vi "Select Item Value.vi"(7 "Section Name":string, 8 "error in (no error)":errorcluster, 10 "Key Name":string, 11 "ODBC-Interface in":refnum<class "ODBC-Interface.lvclass">) -> (0 "error out":errorcluster, 1 "Value":variant, 2 "found":bool, 3 "ODBC-Interface out":refnum<class "ODBC-Interface.lvclass">)   [LabVIEW 2012, in "DB-Configuration.lvlib" / "ODBC-Interface.lvclass"]
doc: "Read item value from database."
uses:
  ODBC-Interface.lvclass
  ODBC-Interface.lvclass/ODBC-Interface.ctl
  <vilib>/addons/database/Connection.llb/Conn Execute.vi
  <vilib>/addons/database/Recordset.llb/Rec Fetch Recordset Data (R).vi
  <vilib>/addons/database/Recordset.llb/Rec Destroy - Connection.vi
  DB-Configuration.lvlib
  <vilib>/addons/database/NI_Database_API.lvlib
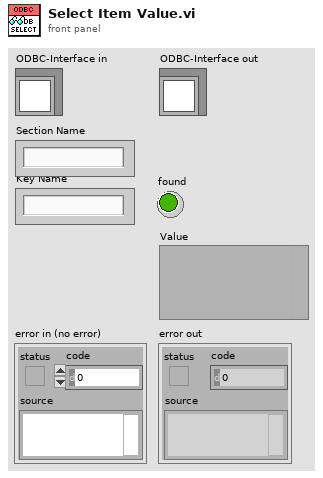
[diagram p1: front panel]
types:
  T1 = typedef "NI_Database_API.lvlib/Conn ObjectReference.ctl" = refnum<k1>
  T2 = typedef "NI_Database_API.lvlib/Rec ObjectReference.ctl" = refnum<k1>
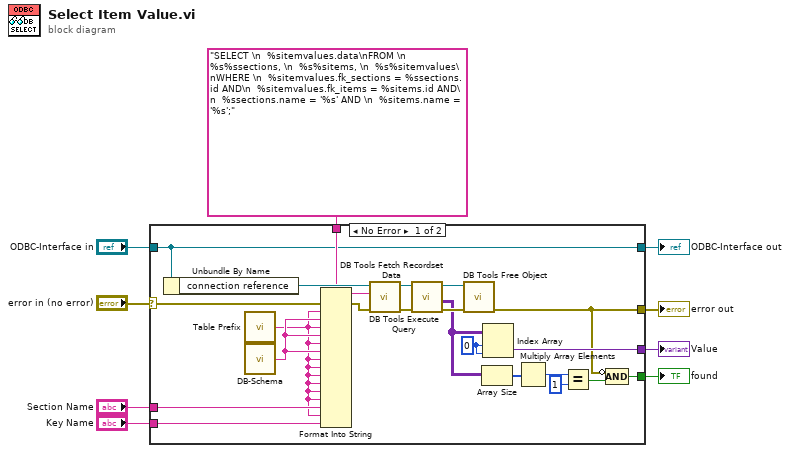
[diagram p0: block diagram]
diagram:
  n1 = case shown="No Error" "error in (no error)" {
    selector: "error in (no error)" -> [w24 w33]
    tunnel: "ODBC-Interface in" -> [w23 w34]
    tunnel: "SELECT \n  %sitemvalues.data\nFROM \n  %s%ssections, \n  %s%sitems, \n  %s%sitemvalues\nWHERE \n  %sitemvalues.fk_sections = %ssections.id AND\n  %sitemvalues.fk_items = %sitems.id AND\n  %ssections.name = '%s' AND \n  %sitems.name = '%s';" -> [w31 _]
    tunnel: [w10 w33] -> w3
    tunnel: [w23 w34] -> w7
    tunnel: "Section Name" -> [w21 _]
    tunnel: "Key Name" -> [w19 _]
    tunnel: [w12 _] -> w2
    tunnel: [w17 _] -> w1
    frame No Error {
      w18 = 0 ("index")
      n2 = Unbundle By Name(w23) -> ("connection reference"=w32:T1)
      n3 = call "Table Prefix.vi"() -> ("DB Table Prefix"=w20:string)
      n4 = call "DB-Schema.vi"() -> ("DB Schema (public.)"=w22:string)
      n5 = Format Into String(format string=w31, error in=w24, w20, w22, w20, w22, w20, w22, w20, w20, w20, w20, w20, w20, w21, w20, w19) -> (resulting string=w30:string, error out=w29:errorcluster)  [unwired: 1 in]
      n6 = call-poly <vilib>:"DB Tools Execute Query.vi"("error in (no error)"=w29, "SQL query"=w30, "connection reference"=w32) -> ("error out"=w27:errorcluster, "recordset reference"=w28:T2)  [unwired: 5 in]
      n7 = call-poly <vilib>:"DB Tools Fetch Recordset Data.vi"("error in (no error)"=w27, "recordset reference"=w28) -> ("error out"=w26:errorcluster, "recordset data"=w16:variant[][], "recordset reference out"=w25:T2)  [unwired: 3 in]
      n8 = call-poly <vilib>:"DB Tools Free Object.vi"("error in (no error)"=w26, "recordset reference"=w25) -> ("error out"=w10:errorcluster)  [unwired: 8 in, 1 out]
      n9 = Array Size(array=w16) -> (size(s)=w15:i32[])
      n10 = Index Array(array=w16, index (row)=w18, index (col)=w18) -> (element=w17:variant)
      n11 = Multiply Array Elements(1:w15) -> (0:w14:i32)
      n12 = Equal?(x=w14, y=1) -> (x = y?=w11:bool)
      n13 = Compound Arithmetic op=AND(invert w10, w11) -> (w12:bool)
    }
    frame Error {
    }
  }
  "error out" <- w3
  "ODBC-Interface out" <- w7
  "Value" <- w1
  "found" <- w2
